vi "synnax writer commit.vi"(8 "error in":errorcluster, 11 "writer":u64) -> (0 "error out":errorcluster, 2 "out_end_ts":i64, 3 "writer out":u64)   [LabVIEW 2026, in "synnax_clib.lvlib"]
doc: "synnax_writer_commit(SynnaxWriter writer, int64_t *out_end_ts, SynnaxError err);"
uses:
  synnax_clib.lvlib
  synnax_clib.dll
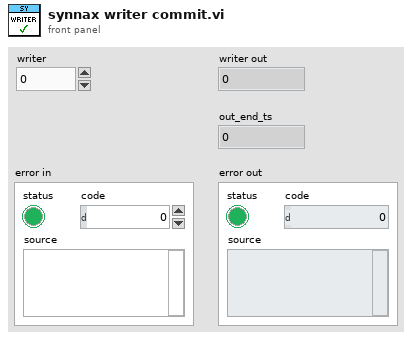
[diagram p1: front panel]
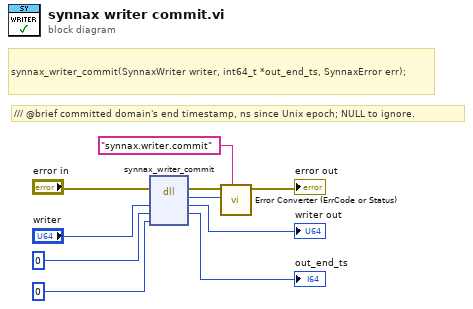
[diagram p0: block diagram]
diagram:
  # "/// @brief committed domain's end timestamp, ns since Unix epoch; NULL to ignore."
  # "synnax_writer_commit(SynnaxWriter writer, int64_t *out_end_ts, SynnaxError err);"
  n1 = dll-call lib="C/synnax/client/labview/lvlib/synnax_clib.*" fn="synnax_writer_commit"(error in="error in", "writer"="writer", "out_end_ts"=i64 0, "err"=u64 0) -> (error out=w5:errorcluster, w4:i32, "writer"=→"writer out":u64, "out_end_ts"=→"out_end_ts":i64)  [unwired: 3 in, 1 out]
  n2 = call "Error Converter (ErrCode or Status).vi"("source"="synnax.writer.commit", "error code"=w4, "error in (no error)"=w5) -> ("error out"=→"error out":errorcluster)  [unwired: 8 in]
